vi "CliColdStart.vi"(0 "ref in":u64, 11 "error in (no error)":errorcluster) -> (4 "ref out":u64, 6 "Result":i32, 15 "error out":errorcluster)   [LabVIEW 2016, in "Snap7.lvlib"]
uses:
  Snap7.lvlib
  win32/lv_snap7.dll
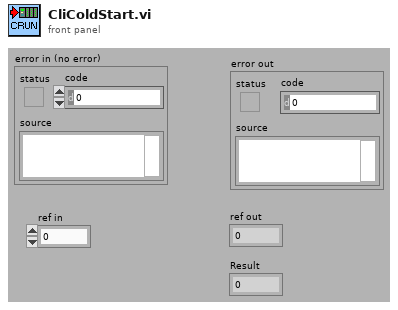
[diagram p1: front panel]
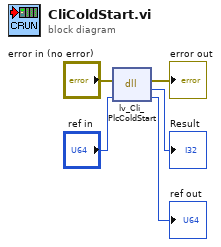
[diagram p0: block diagram]
diagram:
  n1 = dll-call lib="D:/maszup/svn/LineTraceSystem/SOFTWARE/sources/Drivers/PLC/Snap7/lib/win32/lv_snap7.dll" fn="lv_Cli_PlcColdStart"(error in="error in (no error)", "Client"="ref in") -> (error out=→"error out":errorcluster, "return type"=→"Result":i32, "Client"=→"ref out":u64)  [unwired: 2 in, 1 out]
